vi "detector_stop_counter.vi"(8 "error in (no error)":errorcluster, 11 "tt20 in":refnum<class "tt20.lvclass">) -> (0 "error out":errorcluster, 3 "tt20 out":refnum<class "tt20.lvclass">)   [LabVIEW 2015, in "tt20.lvclass"]
uses:
  tt20.lvclass
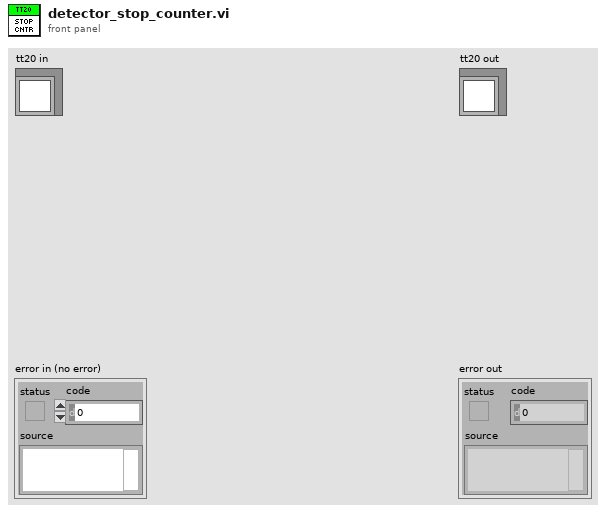
[diagram p1: front panel]
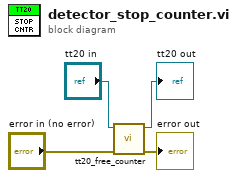
[diagram p0: block diagram]
diagram:
  n1 = call "tt20_free_counter.vi"("error in (no error)"="error in (no error)", "tt20 in"="tt20 in") -> ("error out"=→"error out":errorcluster, "tt20 out"=→"tt20 out":refnum<class "tt20.lvclass">)  [unwired: 8 in]
